vi "Convert Plot Interpolation (List to PN).vi"(8 "Error In":errorcluster, 9 "Plot Interpolation (PN) in":u8, 11 "Plot Interpolation (List)":T1) -> (0 "Error Out":errorcluster, 2 "Plot.Plot Interpolation (PN)":u8)   [LabVIEW 2021, in "Graphs.lvlib"]
uses:
  LabVIEW Plot Interpolation.ctl
  Graphs.lvlib
panel:
  # "see the License on the block diagram (Ctrl+E or Window:Show Block Diagram)"
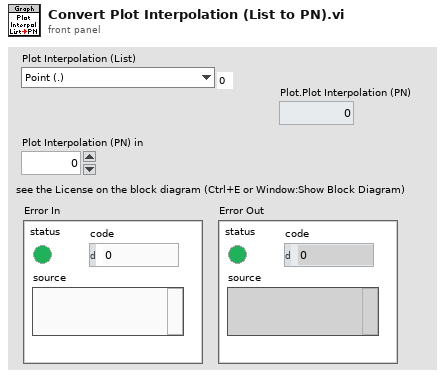
[diagram p1: front panel]
types:
  T1 = typedef "Graphs.lvlib/LabVIEW Plot Interpolation.ctl" = enum16{"Point (.)", "Stepwise Right (--.)", "Line + Point (\\. /)", "Stepwise Left (.--)", "Stepwise Centered (-.-)", "Stepwise Vertical (|.|)", "Line (-)", "Use Previous Plot's Style"}
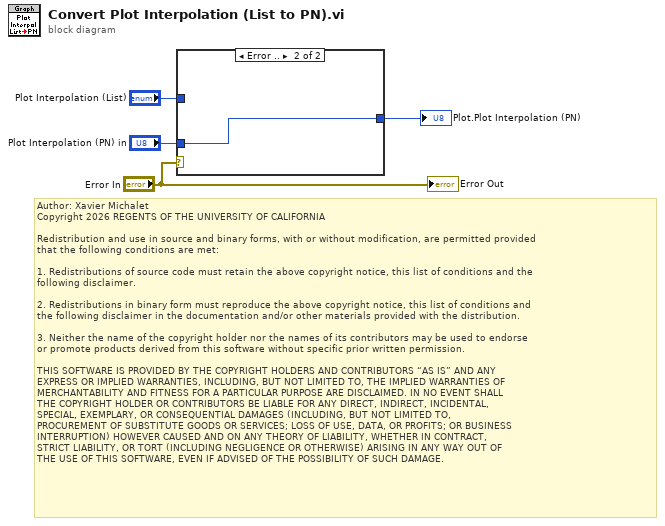
[diagram p0: block diagram]
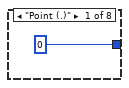
[diagram p3: hidden frame]
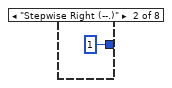
[diagram p4: hidden frame]
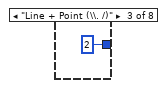
[diagram p5: hidden frame]
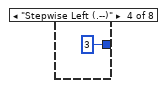
[diagram p6: hidden frame]
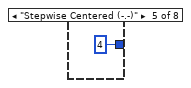
[diagram p7: hidden frame]
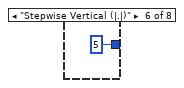
[diagram p8: hidden frame]
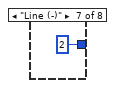
[diagram p9: hidden frame]
diagram:
  # "Author: Xavier Michalet\nCopyright 2026 REGENTS OF THE UNIVERSITY OF CALIFORNIA\n\nRedistribution and use in source and binary forms, with or without modification, are permitted provided\nthat the following conditions are met:\n\n1. Redistributions of source code must retain the above copyright notice, this list of conditions and the\nfollowing disclaimer.\n\n2. Redistributions in binary form must reproduce the above copyright notice, this list of conditions and\nthe following disclaimer in the documentation and/or other materials provided with the distribution.\n\n3. Neither the name of the copyright holder nor the names of its contributors may be used to endorse \nor promote products derived from this software without specific prior written permission.\n\nTHIS SOFTWARE IS PROVIDED BY THE COPYRIGHT HOLDERS AND CONTRIBUTORS “AS IS” AND ANY \nEXPRESS OR IMPLIED WARRANTIES, INCLUDING, BUT NOT LIMITED TO, THE IMPLIED WARRANTIES OF\nMERCHANTABILITY AND FITNESS FOR A PARTICULAR PURPOSE ARE DISCLAIMED. IN NO EVENT SHALL\nTHE COPYRIGHT HOLDER OR CONTRIBUTORS BE LIABLE FOR ANY DIRECT, INDIRECT, INCIDENTAL, \nSPECIAL, EXEMPLARY, OR CONSEQUENTIAL DAMAGES (INCLUDING, BUT NOT LIMITED TO, \nPROCUREMENT OF SUBSTITUTE GOODS OR SERVICES; LOSS OF USE, DATA, OR PROFITS; OR BUSINESS\nINTERRUPTION) HOWEVER CAUSED AND ON ANY THEORY OF LIABILITY, WHETHER IN CONTRACT, \nSTRICT LIABILITY, OR TORT (INCLUDING NEGLIGENCE OR OTHERWISE) ARISING IN ANY WAY OUT OF\nTHE USE OF THIS SOFTWARE, EVEN IF ADVISED OF THE POSSIBILITY OF SUCH DAMAGE."
  n1 = case shown="Error .." "Error In" {
    tunnel: [w7 w16] -> w4
    tunnel: "Plot Interpolation (PN) in" -> [w6 w16]
    tunnel: "Plot Interpolation (List)" -> [w5 _]
    frame No Error {
      n2 = case shown="\"Use Previous Plot's Style\", Default" w5 {
        tunnel: [u8 0 ("Plot.Plot Interpolation") u8 1 ("Plot.Plot Interpolation") u8 2 ("Plot.Plot Interpolation") u8 3 ("Plot.Plot Interpolation") u8 4 ("Plot.Plot Interpolation") u8 5 ("Plot.Plot Interpolation") u8 2 ("Plot.Plot Interpolation") w15] -> w7
        tunnel: w6 -> [_ _ _ _ _ _ _ w15]
        frame "Point (.)" {
        }
        frame "Stepwise Right (--.)" {
        }
        frame "Line + Point (\\. /)" {
        }
        frame "Stepwise Left (.--)" {
        }
        frame "Stepwise Centered (-.-)" {
        }
        frame "Stepwise Vertical (|.|)" {
        }
        frame "Line (-)" {
        }
        frame "Use Previous Plot's Style", Default {
        }
      }
    }
    frame Error {
    }
  }
  "Plot.Plot Interpolation (PN)" <- w4
  "Error Out" <- "Error In"
